vi "pcfs_signal_dither_start.vi"(8 "error in (no error)":errorcluster, 11 "pcfs in":refnum<class "pcfs.lvclass">) -> (0 "error out":errorcluster, 3 "pcfs out":refnum<class "pcfs.lvclass">)   [LabVIEW 2015, in "pcfs.lvclass"]
uses:
  pcfs.lvclass
  pcfs_loop_notifier_tdef.ctl
  pcfs.lvclass/pcfs.ctl
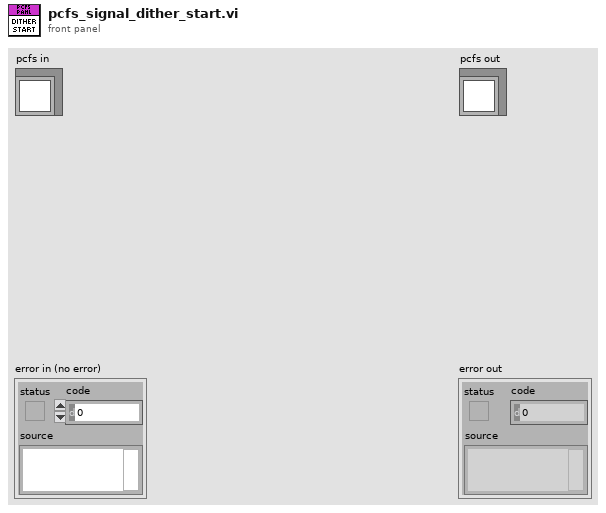
[diagram p1: front panel]
types:
  T1 = typedef "pcfs_loop_notifier_tdef.ctl" = enum16{"exit", "dither", "chart counts"}
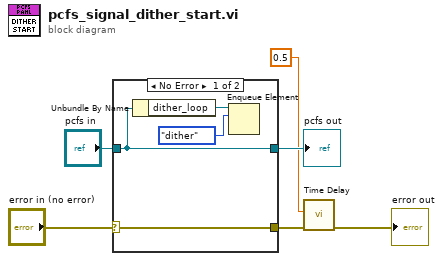
[diagram p0: block diagram]
diagram:
  n1 = case shown="No Error" "error in (no error)" {
    selector: "error in (no error)" -> [w10 w12]
    tunnel: [w10 w12] -> w2
    tunnel: [w9 w11] -> w4
    tunnel: "pcfs in" -> [w9 w11]
    frame No Error {
      n2 = Unbundle By Name(w9) -> ("dither_loop"=w8:refnum<queue>)
      n3 = Enqueue Element(queue=w8, element=pcfs_loop_notifier_tdef."dither") -> ()  [unwired: 2 in, 3 out]
    }
    frame Error {
    }
  }
  "pcfs out" <- w4
  n4 = call "Time Delay"("error in (no error)"=w2, "Delay Time (s)"=0.5) -> ("error out"=→"error out":errorcluster)  [unwired: 9 in]
